vi "Stitch DAQ-scope time.vi"(8 "error in":errorcluster, 9 "Scope Time arrays.Time axis":dbl[](array[numeric]), 10 "DAQ time array (decimated)":dbl[](array[numeric]), 11 "max scope time":dbl) -> (0 "error out":errorcluster, 3 "Stiched scope-DAQ time array":dbl[](array[numeric]))   [LabVIEW 2017, in "Processing.lvlib"]
uses:
  Processing.lvlib
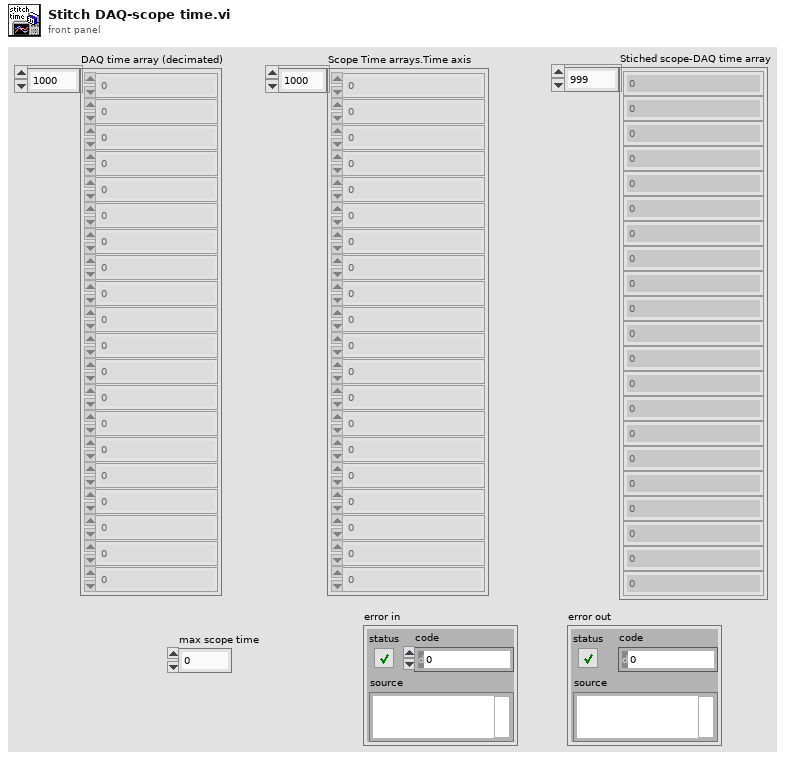
[diagram p1: front panel]
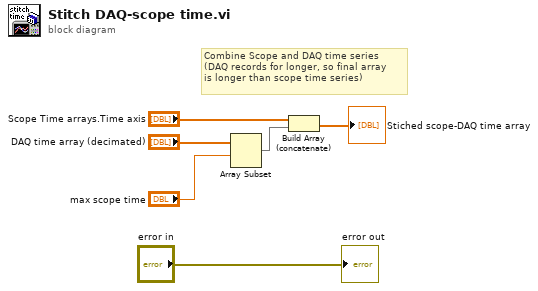
[diagram p0: block diagram]
diagram:
  # "Combine Scope and DAQ time series \n(DAQ records for longer, so final array \nis longer than scope time series)"
  n1 = Array Subset "Array Subset"(array="DAQ time array (decimated)", index="max scope time") -> (w5:dbl[])  [unwired: 1 in]
  n2 = Build Array (concatenate)("Scope Time arrays.Time axis", w5) -> (→"Stiched scope-DAQ time array":dbl[])
  "error out" <- "error in"
